vi "setGrating.vi"(8 "error in (no error)":errorcluster, 9 "Monochromator in":refnum<class "Monochromator.lvclass">, 10 "GratingType":T1=enum."Red", 11 "ReadySate in":refnum<class "ReadySate.lvclass">) -> (0 "error out":errorcluster, 1 "Monochromator out":refnum<class "Monochromator.lvclass">, 3 "ReadySate out":refnum<class "ReadySate.lvclass">)   [LabVIEW 2016, in "ReadySate.lvclass"]
uses:
  ReadySate.lvclass
  Typedefs/GratingType.ctl
  Monochromator/Monochromator.lvclass
  Typedefs/SWStatus.ctl
  Typedefs/AckType.ctl
  Monochromator/Monochromator.lvclass/Monochromator.ctl
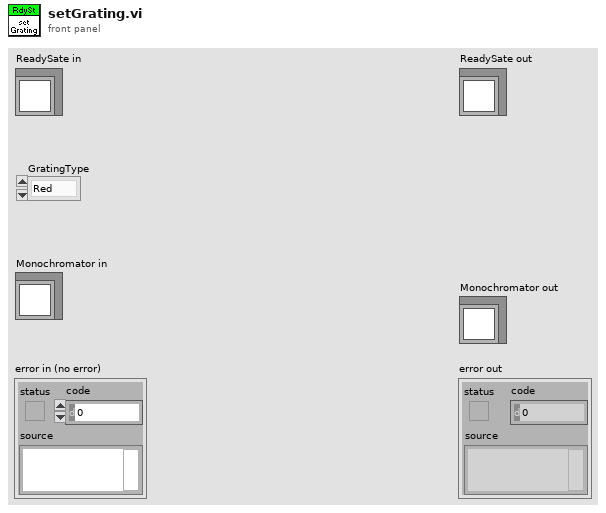
[diagram p1: front panel]
types:
  T1 = typedef "GratingType.ctl" = enum16{"Blue", "Red", "Mirror"}
  T2 = typedef "AckType.ctl" = enum16{"OK", "OutOfRange", "Unknown", "Busy", "Rejected"}
  T3 = typedef "SWStatus.ctl" = enum16{"OfflineState", "ReadyState", "SettingUpState", "FaultState"}
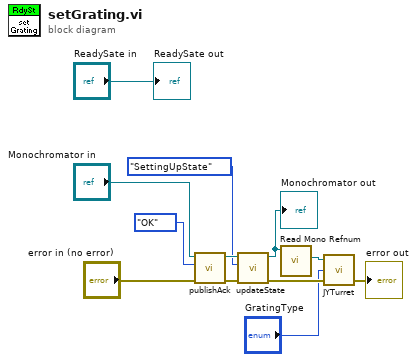
[diagram p0: block diagram]
diagram:
  n1 = call "publishAck.vi"("error in (no error)"="error in (no error)", "Ack"=AckType."OK" ("AckType"), "Monochromator in"="Monochromator in") -> ("error out"=w10:errorcluster, "Monochromator out"=w11:refnum<class "Monochromator.lvclass">)  [unwired: 7 in]
  n2 = call "updateState.vi"("error in (no error)"=w10, "SWStatus"=SWStatus."SettingUpState", "Monochromator in"=w11) -> ("error out"=w6:errorcluster, "Monochromator out"=w7:refnum<class "Monochromator.lvclass">)  [unwired: 7 in]
  "Monochromator out" <- w7
  n3 = call "Read Mono Refnum.vi"("Monochromator in"=w7) -> ("Mono Refnum"=w4:refnum<k7>)  [unwired: 8 in, 2 out]
  n4 = call "JYTurret.vi"("error in (no error)"=w6, "Grating Index"="GratingType", "JYMONOLib.IJYMonoReqd"=w4) -> ("error out"=→"error out":errorcluster)  [unwired: 2 out]
  "ReadySate out" <- "ReadySate in"
